vi "equals.vi"(8 "error in (no error)":errorcluster, 10 "object 2":refnum<class>, 11 "pCircle in":refnum<class "pCircle.lvclass">) -> (0 "error out":errorcluster, 2 "equal?":bool, 3 "pCircle out":refnum<class "pCircle.lvclass">)   [LabVIEW 2018, in "pCircle.lvclass"]
uses:
  pCircle.lvclass
  pCircle.lvclass/pCircle.ctl
  Shape Class/pShape.lvclass
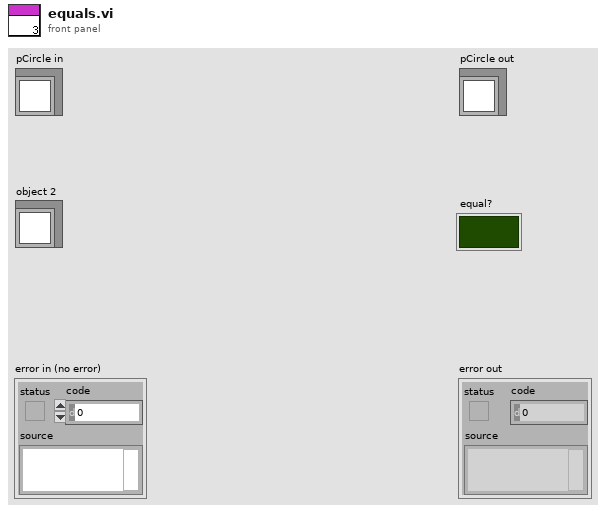
[diagram p1: front panel]
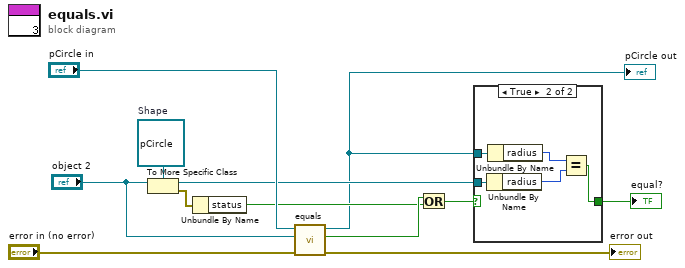
[diagram p0: block diagram]
diagram:
  w9 = refnum<class "pCircle.lvclass"> refnum  # Shape
  n1 = To More Specific Class(target class=w9, reference="object 2") -> (specific class reference=w2:refnum<class "pCircle.lvclass">, error out=w8:errorcluster)  [unwired: 1 in]
  n2 = Unbundle By Name(w8) -> ("status"=w5:bool)
  n3 = call-parent "equals.vi"("error in (no error)"="error in (no error)", "object 2"="object 2", "pShape in"="pCircle in") -> ("error out"=→"error out":errorcluster, "equal?"=w6:bool, "pShape out"=w1:refnum<class "pCircle.lvclass">)  [unwired: 6 in]
  "pCircle out" <- w1
  n4 = Or(x=w6, y=w5) -> (x .or. y?=w4:bool)
  n5 = case shown="True" w4 {
    selector: w4 -> [w13 _]
    tunnel: [w13 w16] -> w3
    tunnel: w2 -> [_ w17]
    tunnel: w1 -> [_ w18]
    frame False {
    }
    frame True {
      n6 = Unbundle By Name(w17) -> ("radius"=w14:i32)
      n7 = Unbundle By Name(w18) -> ("radius"=w15:i32)
      n8 = Equal?(x=w15, y=w14) -> (x = y?=w16:bool)
    }
  }
  "equal?" <- w3
